vi "串口设备参数设置.vi"(8 "布尔文本.文本":string, 9 "section (optional)":string, 10 "监测项描述":string) -> (2 "布尔":bool=TRUE, 3 "输出簇":T2)   [LabVIEW 2016, in "环境动力监测库.lvlib"]
uses:
  <vilib>/Utility/miscctls.llb/LVPointTypeDef.ctl
  <vilib>/Utility/config.llb/NI_LVConfig.lvlib
panel:
  in  "data bits":u64=8 caption="数据比特" min=5 max=8 step=1
  in  "波特率":u64=19200
  in  "停止位":u16(ring)=10 items=["1.0"=10, "1.5"=15, "2.0"=20]
  in  "奇偶校验":u16(ring) items=["None", "Odd", "Even", "Mark", "Space"]
  in  "传感器型号:":T1(ring)
  in  "输入簇":T2
  in  "站号":u64
  in  "返回":bool
  in  "增加":bool
  in  "端口:":T3(ring)
  in  "监测项描述:":string
  # "基本设置"
  # "如:红外XX"
  # "传感器选择"
  # "端口选择"
  # "站号配置"
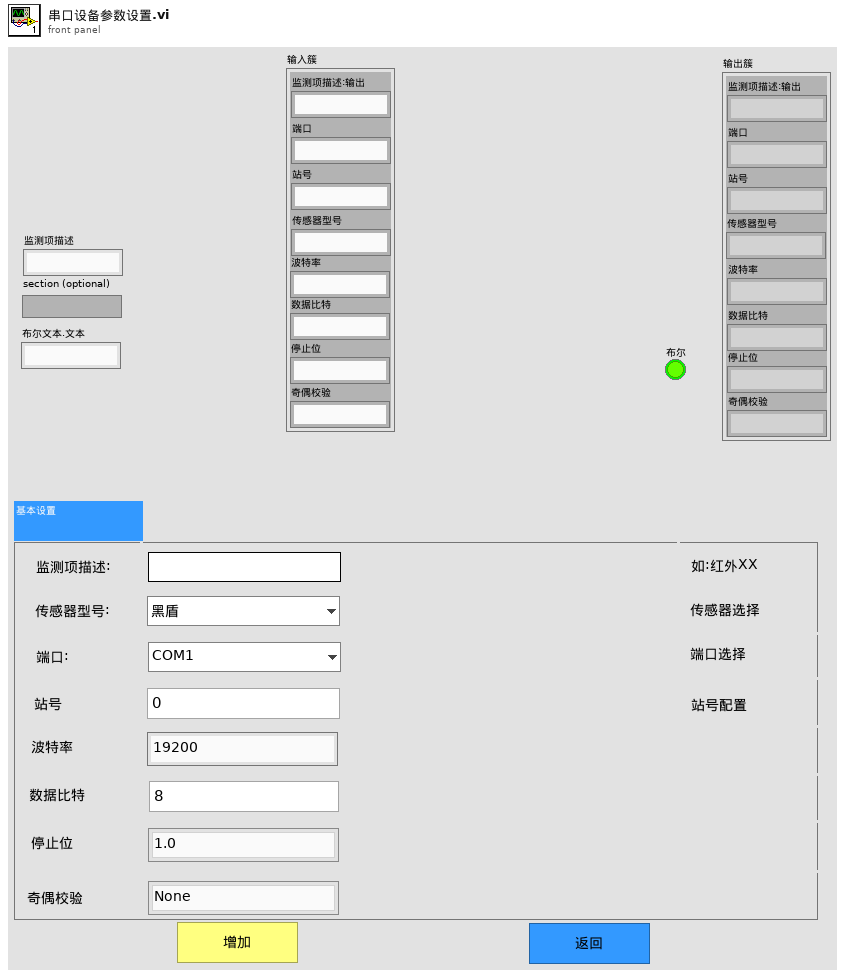
[diagram p1: front panel]
types:
  T1 = enum16{"黑盾", "英维克", "梦幻城堡C6~20KS", "梦幻城堡C1K(S)~C3K(S)"}
  T2 = cluster{"监测项描述:输出":string, "端口":string, "站号":string, "传感器型号":string, "波特率":string, "停止位":string, "奇偶校验":string, "数据比特":string}
  T3 = enum16{"COM1", "COM2", "COM3", "COM4", "COM5", "COM6", "COM7", "COM8", "COM9", "COM10", "COM11", "COM12", "COM13", "COM14", "COM15", "COM16", "COM17", "COM18", "COM19", "COM20"}
  T4 = typedef "LVPointTypeDef.ctl" = cluster{"Horizontal":i16, "Vertical":i16}
  T5 = typedef "NI_LVConfig.lvlib/Config Data RefNum.ctl" = refnum<k1>
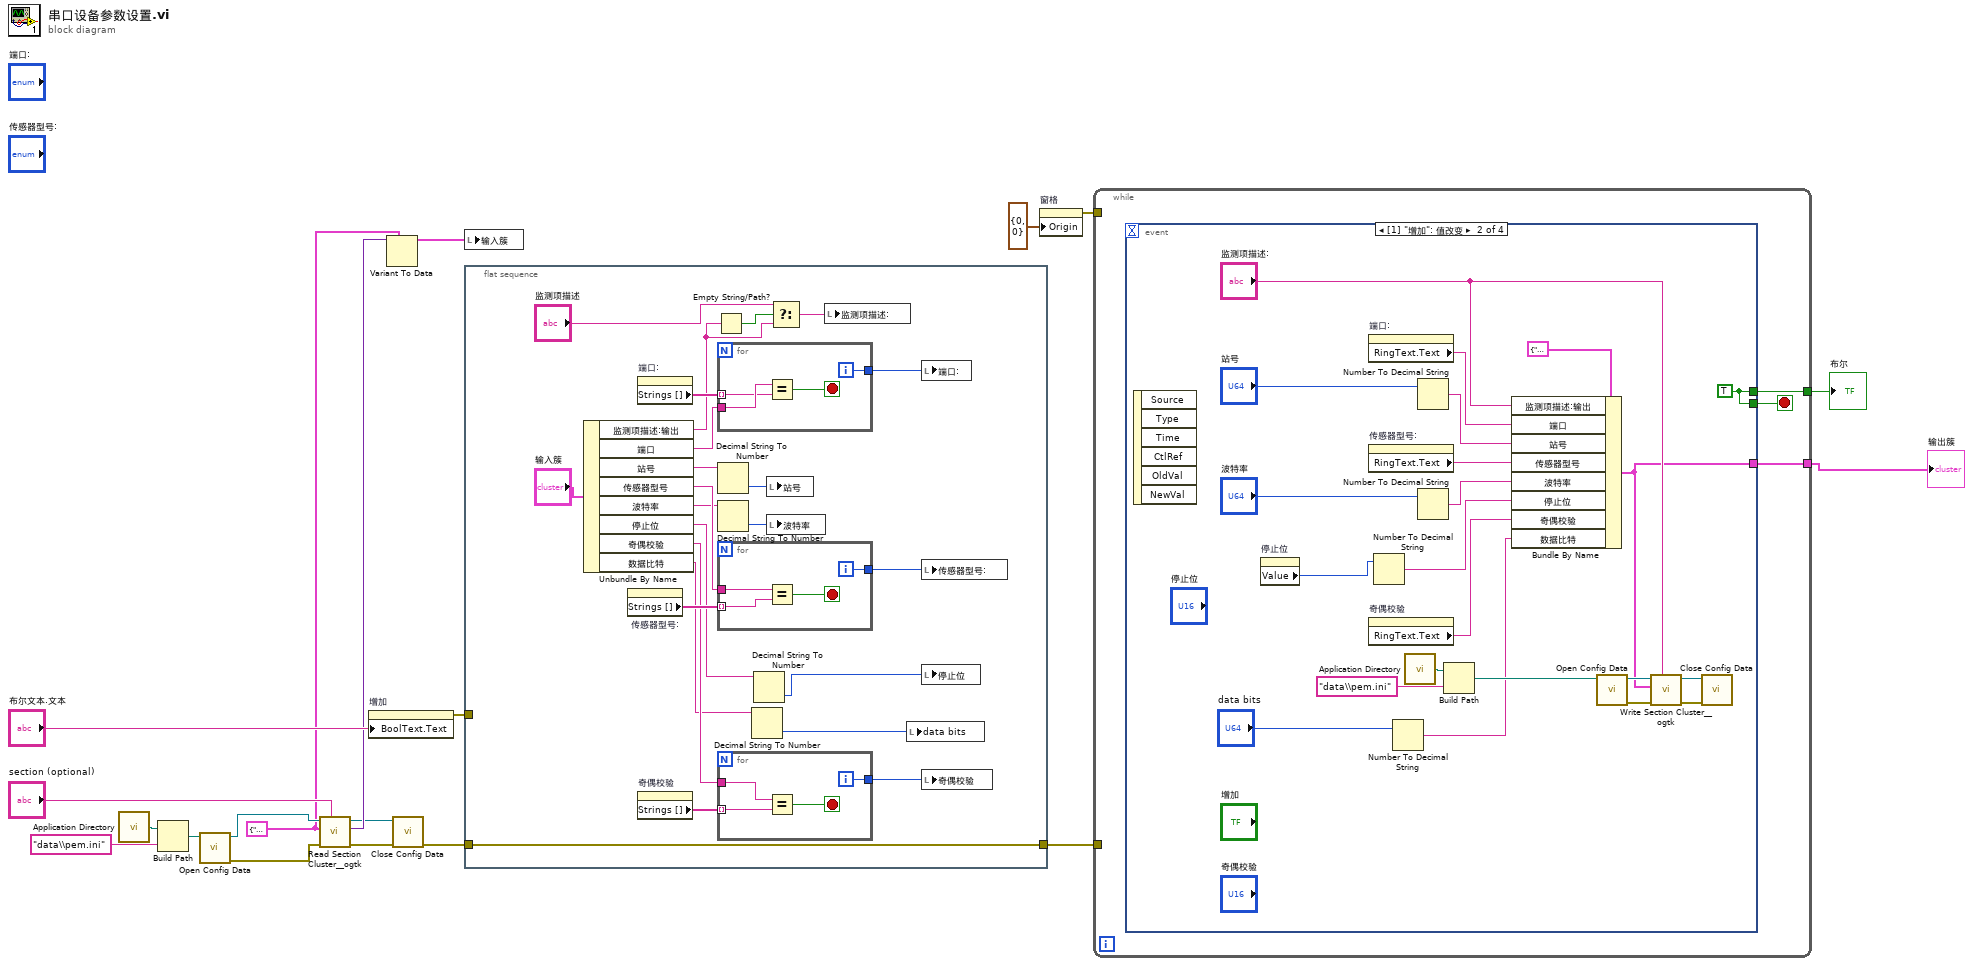
[diagram p0: block diagram]
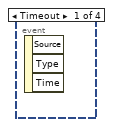
[diagram p2: hidden frame]
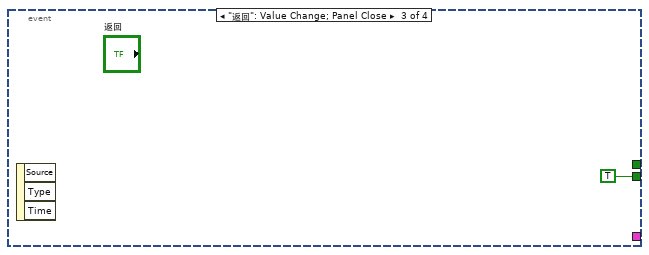
[diagram p3: hidden frame]
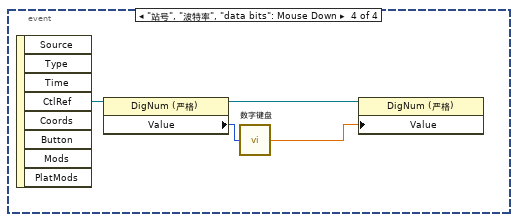
[diagram p4: hidden frame]
diagram:
  w1 = T2 {"监测项描述:输出"="", "端口"="", "站号"="", "传感器型号"="", "波特率"="", "停止位"="", "奇偶校验"="", "数据比特"=""} ("输入簇")
  n1 = call <vilib>:"Application Directory.vi"() -> ("Application Directory"=w12:path)
  n2 = Build Path(base path=w12, name or relative path="data\\pem.ini" ("名称或相对路径")) -> (appended path=w13:path)
  n3 = call <vilib>:"Open Config Data.vi"("configuration file path"=w13) -> ("error out"=w14:errorcluster, "refnum"=w15:T5)  [unwired: 8 in, 1 out]
  n4 = call <userlib>:"Read Section Cluster__ogtk.vi"("section (optional)"="section (optional)", "error in (no error)"=w14, "Section Formatted Cluster Type"=w1, "refnum"=w15) -> ("error out"=w6:errorcluster, "Section Formatted Cluster"=w9:variant, "dup refnum"=w7:T5)  [unwired: 3 in, 2 out]
  n5 = property on="增加" class="Bool"("BoolText.Text"="布尔文本.文本") -> (error out=w5:errorcluster)  [unwired: 2 in, 1 out]
  n6 = Variant To Data(type=w1, Variant=w9) -> (data=w8:T2)  [unwired: 1 in, 1 out]
  n7 = call <vilib>:"Close Config Data.vi"("error in (no error)"=w6, "refnum"=w7) -> ("error out"=w4:errorcluster)  [unwired: 8 in, 1 out]
  n8 = local write "输入簇"(w8) -> ()
  n9 = flat-sequence {
    tunnel: w5 -> [_]
    tunnel: w4 -> [w37]
    tunnel: [w37] -> w3
    frame #0 {
      n10 = Unbundle By Name("输入簇") -> ("监测项描述:输出"=w34:string, "端口"=w41:string, "站号"=w38:string, "传感器型号"=w30:string, "波特率"=w27:string, "停止位"=w23:string, "奇偶校验"=w24:string, "数据比特"=w21:string)
      n11 = property on="传感器型号:" class="Enum (严格)"() -> ("Strings []"=w31:string[])  [unwired: 2 in, 2 out]
      n12 = property on="端口:" class="Enum (严格)"() -> ("Strings []"=w40:string[])  [unwired: 2 in, 2 out]
      n13 = property on="奇偶校验" class="Ring (严格)"() -> ("Strings []"=w25:string[])  [unwired: 2 in, 2 out]
      n14 = Empty String/Path?(string/path=w34) -> (empty?=w36:bool)
      n15 = for {
        tunnel: w41 -> [w54]
        tunnel: [w52] -> w39
        tunnel: w40 -> [w51] mode=indexing
        i -> [w52]
        stop <- w53 stop-if-true
        n16 = Equal?(x=w54, y=w51) -> (x = y?=w53:bool)
      }
      n17 = Decimal String To Number(string=w38) -> (number=w32:i32)  [unwired: 2 in, 1 out]
      n18 = Decimal String To Number(string=w27) -> (number=w28:i32)  [unwired: 2 in, 1 out]
      n19 = for {
        tunnel: w30 -> [w50]
        tunnel: [w48] -> w29
        tunnel: w31 -> [w47] mode=indexing
        i -> [w48]
        stop <- w49 stop-if-true
        n20 = Equal?(x=w50, y=w47) -> (x = y?=w49:bool)
      }
      n21 = for {
        tunnel: w24 -> [w46]
        tunnel: [w44] -> w26
        tunnel: w25 -> [w43] mode=indexing
        i -> [w44]
        stop <- w45 stop-if-true
        n22 = Equal?(x=w46, y=w43) -> (x = y?=w45:bool)
      }
      n23 = Decimal String To Number(string=w21) -> (number=w20:i32)  [unwired: 2 in, 1 out]
      n24 = Decimal String To Number(string=w23) -> (number=w22:i32)  [unwired: 2 in, 1 out]
      n25 = local write "站号"(w32) -> ()
      n26 = local write "波特率"(w28) -> ()
      n27 = Select(t="监测项描述", s=w36, f=w34) -> (s? t:f=w33:string)
      n28 = local write "监测项描述:"(w33) -> ()
      n29 = local write "data bits"(w20) -> ()
      n30 = local write "端口:"(w39) -> ()
      n31 = local write "传感器型号:"(w29) -> ()
      n32 = local write "停止位"(w22) -> ()
      n33 = local write "奇偶校验"(w26) -> ()
    }
  }
  n34 = property on="窗格" class="Pane"("Origin"=T4 {"Horizontal"=0, "Vertical"=0} ("原点")) -> (error out=w19:errorcluster)  [unwired: 2 in, 1 out]
  n35 = while {
    tunnel: w19 -> [_]
    tunnel: [w57] -> w2
    tunnel: [w55] -> w17
    tunnel: w3 -> [_]
    stop <- w56 stop-if-true
    n36 = event shown="[1] \"增加\": 值改变" {
      selector: _ -> [_ _ _ _]
      dyn-events: _ -> [_ _ _ _]
      timeout: _ -> [_ _ _ _]
      tunnel: [_ w71 _ _] -> w57
      tunnel: [_ w70 TRUE _] -> w56
      tunnel: [_ w70 _ _] -> w55
      event Timeout {
        n37 = event-data() -> ()  [unwired: 1 in, 3 out]
      }
      event "增加": Value Change {
        w70 = TRUE
        n38 = event-data() -> ()  [unwired: 1 in, 6 out]
        n39 = property on="停止位" class="Ring (严格)"() -> ("Value"=w62:u16)  [unwired: 2 in, 2 out]
        n40 = property on="端口:" class="Enum (严格)"() -> ("RingText.Text"=w69:string)  [unwired: 2 in, 2 out]
        n41 = property on="传感器型号:" class="Enum (严格)"() -> ("RingText.Text"=w66:string)  [unwired: 2 in, 2 out]
        n42 = property on="奇偶校验" class="Ring (严格)"() -> ("RingText.Text"=w63:string)  [unwired: 2 in, 2 out]
        n43 = Number To Decimal String(number=w62) -> (decimal integer string=w61:string)  [unwired: 1 in]
        n44 = Number To Decimal String(number="data bits") -> (decimal integer string=w59:string)  [unwired: 1 in]
        n45 = call <vilib>:"Application Directory.vi"() -> ("Application Directory"=w76:path)
        n46 = Number To Decimal String(number="站号") -> (decimal integer string=w68:string)  [unwired: 1 in]
        n47 = Number To Decimal String(number="波特率") -> (decimal integer string=w64:string)  [unwired: 1 in]
        n48 = Build Path(base path=w76, name or relative path="data\\pem.ini" ("名称或相对路径")) -> (appended path=w77:path)
        n49 = Bundle By Name(cluster=T2 {"监测项描述:输出"="", "端口"="", "站号"="", "传感器型号"="", "波特率"="", "停止位"="", "奇偶校验"="", "数据比特"=""} ("输出簇"), "监测项描述:输出"="监测项描述:", "端口"=w69, "站号"=w68, "传感器型号"=w66, "波特率"=w64, "停止位"=w61, "奇偶校验"=w63, "数据比特"=w59) -> (w71:T2)
        n50 = call <vilib>:"Open Config Data.vi"("configuration file path"=w77) -> ("error out"=w78:errorcluster, "refnum"=w79:T5)  [unwired: 8 in, 1 out]
        n51 = call <userlib>:"Write Section Cluster__ogtk.vi"("section (optional)"="监测项描述:", "error in (no error)"=w78, "Section Formatted Cluster"=w71, "refnum"=w79) -> ("error out"=w72:errorcluster, "dup refnum"=w73:T5)  [unwired: 6 in]
        n52 = call <vilib>:"Close Config Data.vi"("error in (no error)"=w72, "refnum"=w73) -> ()  [unwired: 8 in, 2 out]
      }
      event "返回": Value Change; Panel Close {
        n53 = event-data() -> ()  [unwired: 1 in, 3 out]
      }
      event "站号", "波特率", "data bits": Mouse Down {
        n54 = event-data() -> ("CtlRef"=w84:refnum<vi>)  [unwired: 1 in, 7 out]
        n55 = property class="DigNum (严格)"(reference=w84) -> (reference out=w82:refnum<vi>, "Value"=w83:u64)  [unwired: 1 in, 1 out]
        n56 = call "数字键盘.vi"("OldNumber"=w83) -> ("NewNumber"=w81:sgl)
        n57 = property class="DigNum (严格)"(reference=w82, "Value"=w81) -> ()  [unwired: 1 in, 2 out]
      }
    }
  }
  "输出簇" <- w2
  "布尔" <- w17
